vi "Get TE and Task Name.vi"(8 "error in (no error)":errorcluster, 11 "DAQ Actor in":refnum<class "DAQ Actor.lvclass">) -> (0 "error out":errorcluster, 1 "Task Name":string, 2 "TimingEngine":T1, 3 "DAQ Actor out":refnum<class "DAQ Actor.lvclass">)   [LabVIEW 2018, in "Data Acquisition.lvlib" / "DAQ Actor.lvclass"]
uses:
  DAQ Actor.lvclass
  Common/Controls/TE_Designator.ctl
  DAQ Actor.lvclass/DAQ Actor.ctl
  Class DAQ Task/DAQ Task.lvclass/DAQ Task.ctl
  Class DAQ Task/Read Task Name.vi
  Class DAQ Task/DAQ Task.lvclass
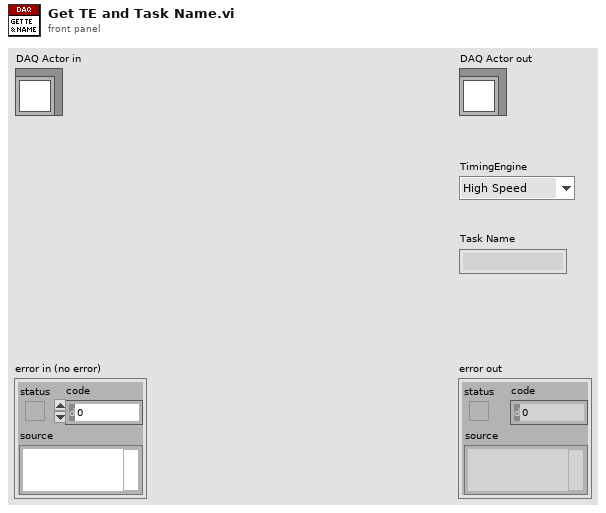
[diagram p1: front panel]
types:
  T1 = typedef "TE_Designator.ctl" = enum16{"High Speed", "Low Speed"}
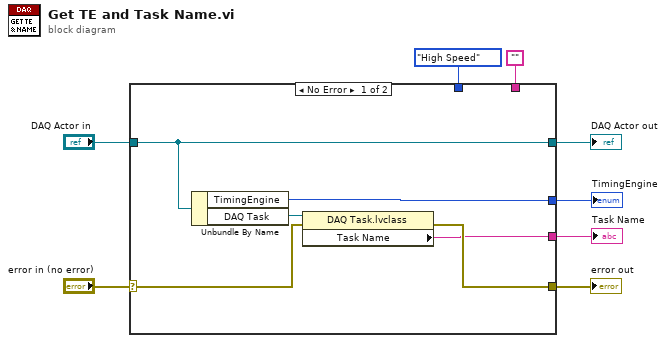
[diagram p0: block diagram]
diagram:
  n1 = case shown="No Error" "error in (no error)" {
    selector: "error in (no error)" -> [w12 w18]
    tunnel: [w10 w18] -> w7
    tunnel: [w14 w17] -> w5
    tunnel: "DAQ Actor in" -> [w14 w17]
    tunnel: [w11 w15] -> w4
    tunnel: [w9 w16] -> w3
    tunnel: "" -> [_ w16]
    tunnel: TE_Designator."High Speed" ("TimingEngine") -> [_ w15]
    frame No Error {
      n2 = Unbundle By Name(w14) -> ("TimingEngine"=w11:T1, "DAQ Task"=w13:refnum<class "DAQ Task.lvclass">)
      n3 = property class="DAQ Task.lvclass"(reference=w13, error in=w12) -> (error out=w10:errorcluster, "Task Name"=w9:string)  [unwired: 1 out]
    }
    frame Error {
    }
  }
  "error out" <- w7
  "DAQ Actor out" <- w5
  "TimingEngine" <- w4
  "Task Name" <- w3
